vi "GetPluginType.vi"(7 "reference":refnum<vi>, 8 "ErrorArray In":errorcluster[](array[cluster]), 10 "IniFilePaths":path[](array[path]), 11 "Instrument Modules In":T1=[{"PluginSelection"=4, "ConfigDialog"=FALSE}]) -> (0 "ErrorArray Out":errorcluster[](array[cluster]), 2 "Instrument Modules Out":T1=[{"PluginSelection"=4, "ConfigDialog"=FALSE}], 3 "PluginTypes":string[](array[string]))   [LabVIEW 2018]
doc: "This VI extracts the plugin type from the configuration ini file."
uses:
  Framework/InstrumentModulesControl.ctl
  <vilib>/Utility/config.llb/Read Key (String).vi
  <vilib>/Utility/error.llb/Error Cluster From Error Code.vi
  <vilib>/ErrorRing/Error Ring.xnode
  LV_Ini/Ini_lib.lvlib
  <userlib>/NIST/NISTErrorLib/NISTErrorLib.lvlib
  <vilib>/Utility/config.llb/NI_LVConfig.lvlib
panel:
  out "logical OR":bool
  out "x = y?":bool[](array[boolean])
  out "PluginTypes":string[](array[string])
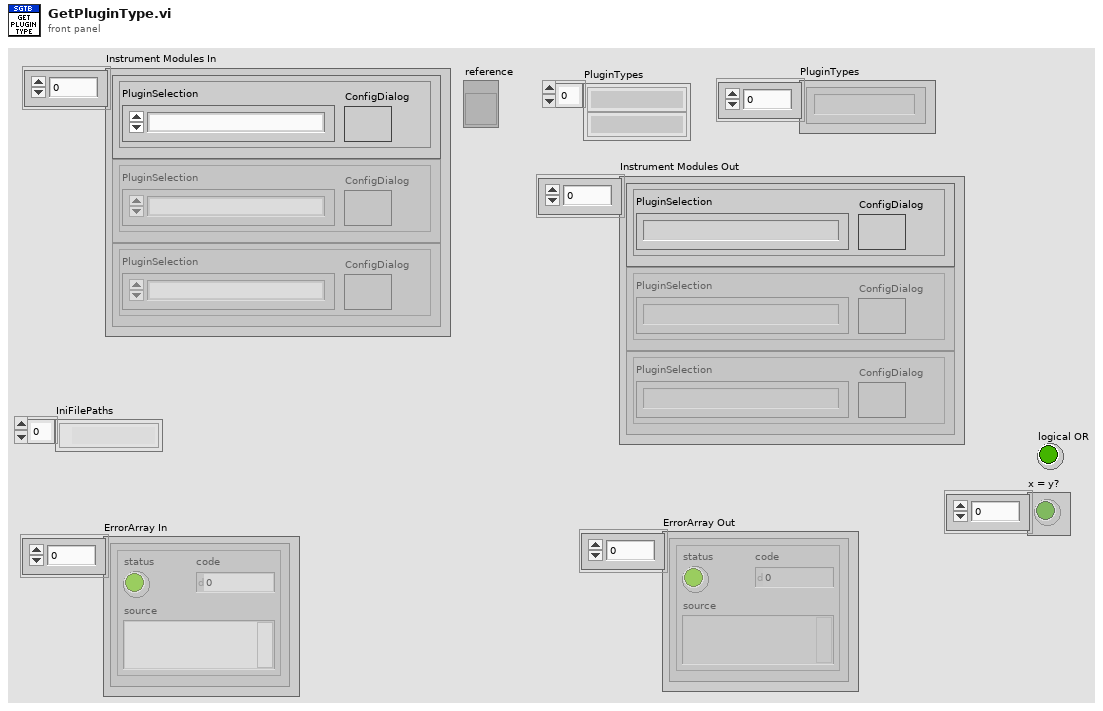
[diagram p1: front panel]
types:
  T1 = typedef "InstrumentModulesControl.ctl" = cluster{"PluginSelection":u16, "ConfigDialog":bool}[]
  T2 = typedef "NI_LVConfig.lvlib/Config Data RefNum.ctl" = refnum<k1>
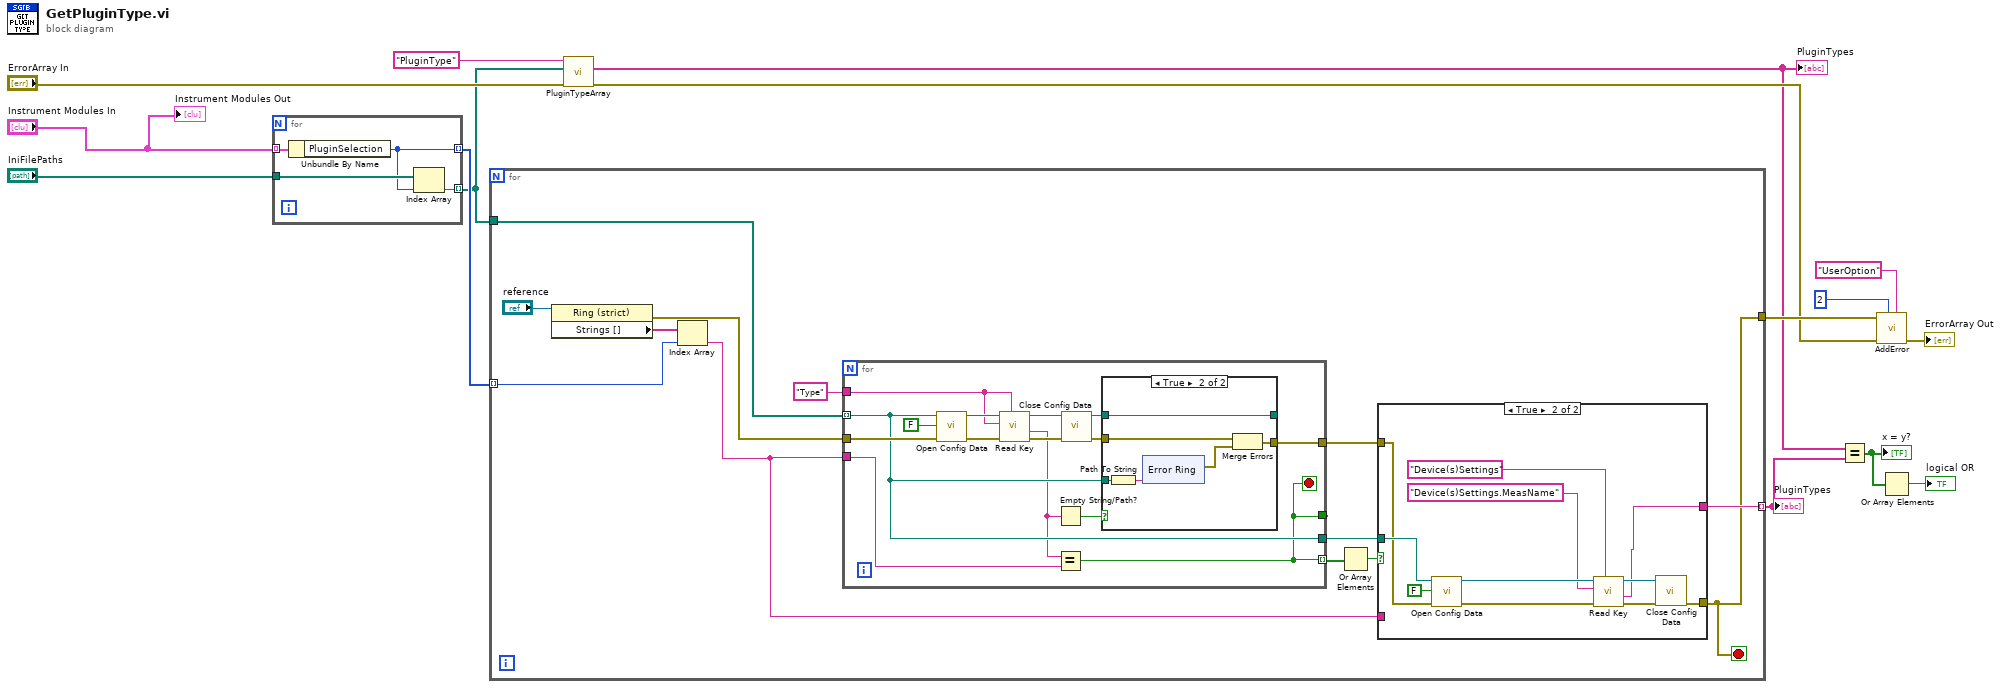
[diagram p0: block diagram]
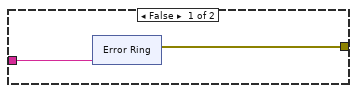
[diagram p3: hidden frame]
diagram:
  n1 = for {
    tunnel: "Instrument Modules In" -> [w19] mode=indexing
    tunnel: "IniFilePaths" -> [w18]
    tunnel: [w17] -> w5 mode=indexing
    tunnel: [w16] -> w6 mode=indexing
    n2 = Unbundle By Name(w19) -> ("PluginSelection"=w16:u16)
    n3 = Index Array(array=w18, index=w16) -> (element=w17:path)
  }
  n4 = for {
    tunnel: [w21] -> w10
    tunnel: w6 -> [w30] mode=indexing
    tunnel: w5 -> [w25]
    tunnel: [w22] -> w4 mode=indexing
    stop <- w21 stop-if-true
    n5 = property class="Ring (strict)"(reference="reference") -> (error out=w24:errorcluster, "Strings []"=w32:string[])  [unwired: 1 in, 1 out]
    n6 = Index Array(array=w32, index=w30) -> (element=w23:string)
    n7 = for {
      tunnel: w25 -> [w36] mode=indexing
      tunnel: "Type" ("section") -> [w40]
      tunnel: w23 -> [w34]
      tunnel: [w38] -> w28
      tunnel: w24 -> [w37]
      tunnel: [w36] -> w29
      tunnel: [w33] -> _
      tunnel: [w33] -> w27 mode=indexing
      stop <- w33 stop-if-true
      n8 = call <vilib>:"Open Config Data.vi"("error in (no error)"=w37, "create file if necessary (T)"=FALSE, "configuration file path"=w36) -> ("error out"=w46:errorcluster, "refnum"=w45:T2)  [unwired: 6 in, 1 out]
      n9 = call-poly <vilib>:"Read Key.vi"("section"=w40, "error in (no error)"=w46, "key"=w40, "refnum"=w45) -> ("error out"=w43:errorcluster, "value"=w35:string, "refnum out"=w44:T2)  [unwired: 4 in, 1 out]
      n10 = Empty String/Path?(string/path=w35) -> (empty?=w42:bool)
      n11 = Equal?(x=w35, y=w34) -> (x = y?=w33:bool)
      n12 = call <vilib>:"Close Config Data.vi"("error in (no error)"=w43, "refnum"=w44) -> ("error out"=w41:errorcluster, "file path"=w39:path)  [unwired: 8 in]
      n13 = case shown="True" w42 {
        tunnel: w41 -> [w49 w54]
        tunnel: [w49 w53] -> w38
        tunnel: w36 -> [_ w51]
        tunnel: w39 -> [w48 w50]
        tunnel: [w48 w50] -> _
        frame False {
        }
        frame True {
          n14 = Path To String(path=w51) -> (string=w52:string)
          n15 = xnode "Error Ring"("parameter 0"=w52) -> ("error out"=w55:errorcluster)
          n16 = Merge Errors(w54, w55) -> (w53:errorcluster)
        }
      }
    }
    n17 = Or Array Elements(Boolean array=w27) -> (logical OR=w26:bool)
    n18 = case shown="True" w26 {
      tunnel: w29 -> [_ w77]
      tunnel: w28 -> [_ w73]
      tunnel: [w64 w71] -> w21
      tunnel: w23 -> [w63 _]
      tunnel: [_ w70] -> w22
      frame False {
        n19 = xnode ("Error Ring")("parameter 0"=w63) -> ("error out"=w64:errorcluster)
      }
      frame True {
        n20 = call <vilib>:"Open Config Data.vi"("error in (no error)"=w73, "create file if necessary (T)"=FALSE, "configuration file path"=w77) -> ("error out"=w79:errorcluster, "refnum"=w80:T2)  [unwired: 6 in, 1 out]
        n21 = call-poly <vilib>:"Read Key.vi"("section"="Device(s)Settings", "error in (no error)"=w79, "key"="Device(s)Settings.MeasName" ("section"), "refnum"=w80) -> ("error out"=w76:errorcluster, "value"=w70:string, "refnum out"=w75:T2)  [unwired: 4 in, 1 out]
        n22 = call <vilib>:"Close Config Data.vi"("error in (no error)"=w76, "refnum"=w75) -> ("error out"=w71:errorcluster)  [unwired: 8 in, 1 out]
      }
    }
  }
  "PluginTypes" <- w4
  n23 = call "PluginTypeArray.vi"("ErrorArray Out in"="ErrorArray In", "INIFilePaths"=w5, "section"="PluginType") -> ("ErrorArray Out out"=w8:errorcluster[], "PluginTypes"=w3:string[])  [unwired: 6 in, 1 out]
  "PluginTypes" <- w3
  n24 = Equal?(x=w3, y=w4) -> (x = y?=w2:bool[])
  "x = y?" <- w2
  n25 = call <userlib>:"AddError.vi"("Severity"="UserOption", "Priority"=u8 2, "ErrorArray"=w8, "error in (no error)"=w10) -> ("ErrorArray"=→"ErrorArray Out":errorcluster[])  [unwired: 6 in, 1 out]
  n26 = Or Array Elements(Boolean array=w2) -> (logical OR=→"logical OR":bool)
  "Instrument Modules Out" <- "Instrument Modules In"
